vi "Count Matched Requirements.vi"(7 "test":T1, 9 "Total":u32, 11 "Matrix":bool[][](array[boolean])) -> (0 "Pct":dbl, 2 "Nb Requirements":u32)   [LabVIEW 2021, in "Bananas.lvlib" / "Pips.lvclass"]
uses:
  Pips.lvclass
  row_col_test -- enum.ctl
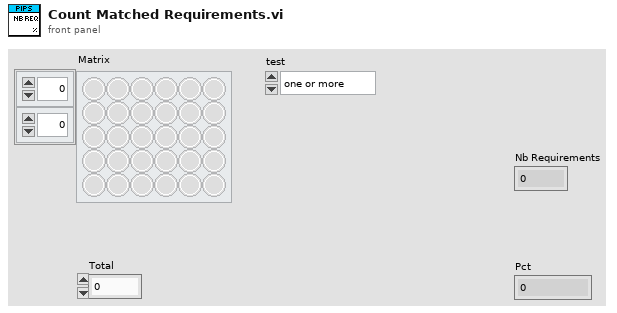
[diagram p1: front panel]
types:
  T1 = typedef "Bananas.lvlib/Pips.lvclass/row_col_test -- enum.ctl" = enum16{"one or more", "all", "none"}
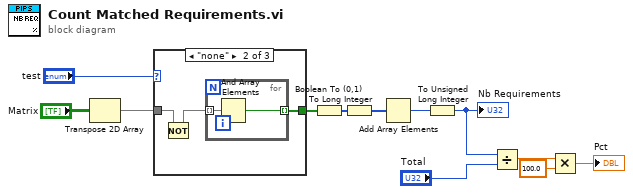
[diagram p0: block diagram]
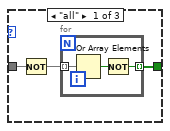
[diagram p2: hidden frame]
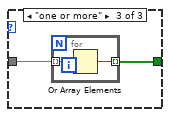
[diagram p3: hidden frame]
diagram:
  n1 = Transpose 2D Array(2D array="Matrix") -> (transposed array=w7:bool[][])
  n2 = case shown="\"none\"" "test" {
    tunnel: [w15 w21 w25] -> w8
    tunnel: w7 -> [w14 w19 w24]
    frame "all" {
      n3 = Not(x=w14) -> (.not. x?=w13:bool[][])
      n4 = for {
        tunnel: w13 -> [w18] mode=indexing
        tunnel: [w16] -> w15 mode=indexing
        n5 = Or Array Elements(Boolean array=w18) -> (logical OR=w17:bool)
        n6 = Not(x=w17) -> (.not. x?=w16:bool)
      }
    }
    frame "none" {
      n7 = Not(x=w19) -> (.not. x?=w20:bool[][])
      n8 = for {
        tunnel: w20 -> [w23] mode=indexing
        tunnel: [w22] -> w21 mode=indexing
        n9 = And Array Elements(Boolean array=w23) -> (logical AND=w22:bool)
      }
    }
    frame "one or more" {
      n10 = for {
        tunnel: w24 -> [w27] mode=indexing
        tunnel: [w26] -> w25 mode=indexing
        n11 = Or Array Elements(Boolean array=w27) -> (logical OR=w26:bool)
      }
    }
  }
  n12 = Boolean To (0,1)(Boolean=w8) -> (0, 1=w9:i16[])
  n13 = To Long Integer(number=w9) -> (32bit integer=w10:i32[])
  n14 = Add Array Elements(numeric array=w10) -> (sum=w12:i32)
  n15 = To Unsigned Long Integer(number=w12) -> (unsigned 32bit integer=w3:u32)
  "Nb Requirements" <- w3
  n16 = Divide(x=w3, y="Total") -> (x/y=w5:dbl)
  n17 = Multiply(x=w5, y=100.0) -> (x*y=→"Pct":dbl)
